vi "PID.vi"(0 "Set Point":dbl(knob)=0.6 scale=0.5..1.0, 1 "Min output value":dbl=0.5, 2 "Max output value":dbl=1.0, 3 "dt":dbl=0.01, 5 "Process Variable":dbl, 7 "Previous Output":dbl, 9 "Previous Error":dbl, 11 "Previous Integral":dbl, 12 "Proportional Gain":dbl, 13 "Integral Gain":dbl, 14 "Derivative Gain":dbl) -> (6 "Output":dbl, 10 "Current Error":dbl, 15 "Integral Error":dbl)   [LabVIEW 2012, in "Pressure Regulator Controller.lvlib"]
uses:
  Pressure Regulator Controller.lvlib
panel:
  in  "PID":enum32{"Main", "Settings", "Errors"}(tab)
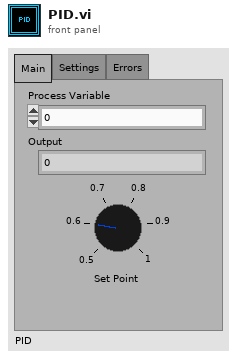
[diagram p1: front panel]
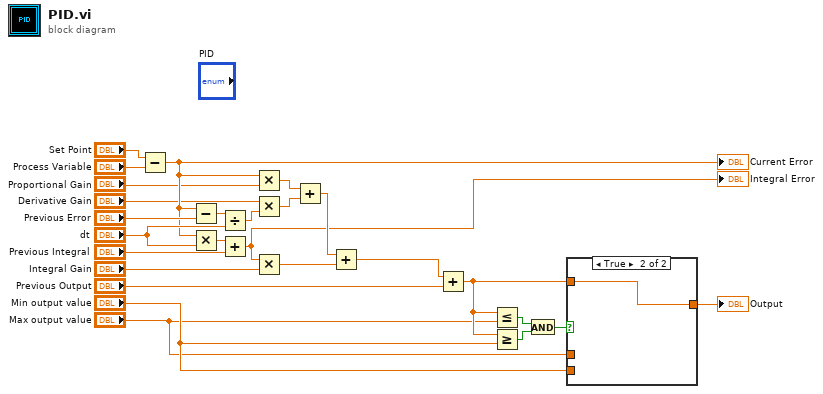
[diagram p0: block diagram]
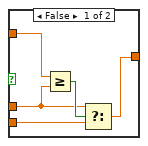
[diagram p2: hidden frame]
diagram:
  n1 = Subtract(x="Set Point", y="Process Variable") -> (x-y=w17:dbl)
  "Current Error" <- w17
  n2 = Subtract(x=w17, y="Previous Error") -> (x-y=w20:dbl)
  n3 = Multiply(x=w17, y="dt") -> (x*y=w23:dbl)
  n4 = Divide(x=w20, y="dt") -> (x/y=w15:dbl)
  n5 = Add(x=w23, y="Previous Integral") -> (x+y=w9:dbl)
  "Integral Error" <- w9
  n6 = Multiply(x=w17, y="Proportional Gain") -> (x*y=w13:dbl)
  n7 = Multiply(x="Derivative Gain", y=w15) -> (x*y=w12:dbl)
  n8 = Multiply(x=w9, y="Integral Gain") -> (x*y=w10:dbl)
  n9 = Add(x=w13, y=w12) -> (x+y=w11:dbl)
  n10 = Add(x=w11, y=w10) -> (x+y=w6:dbl)
  n11 = Add(x=w6, y="Previous Output") -> (x+y=w5:dbl)
  n12 = Less Or Equal?(x=w5, y="Max output value") -> (x <= y?=w26:bool)
  n13 = Greater Or Equal?(x=w5, y="Min output value") -> (x >= y?=w25:bool)
  n14 = And(x=w26, y=w25) -> (x .and. y?=w24:bool)
  n15 = case shown="True" w24 {
    tunnel: w5 -> [w31 w32]
    tunnel: "Min output value" -> [w29 _]
    tunnel: "Max output value" -> [w28 _]
    tunnel: [w27 w32] -> w8
    frame False {
      n16 = Greater Or Equal?(x=w31, y=w28) -> (x >= y?=w30:bool)
      n17 = Select(t=w28, s=w30, f=w29) -> (s? t:f=w27:dbl)
    }
    frame True {
    }
  }
  "Output" <- w8
